vi "USB-HID-LabVIEW.vi"() -> ()   [LabVIEW 2016]
uses:
  <vilib>/Instr/_visa.llb/Select Event Type.ctl
panel:
  out "VISA resource name 2":refnum<visa-resource-name>
  out "error out":errorcluster
  out "string":string
  out "element":u8
  out "unsigned 8bit integer":u8[](array[numeric])
  out "status":bool
  in  "timeout (0)":u32
  in  "number":u8
  in  "error in (no error)":errorcluster
  in  "VISA resource name":refnum<visa-resource-name>
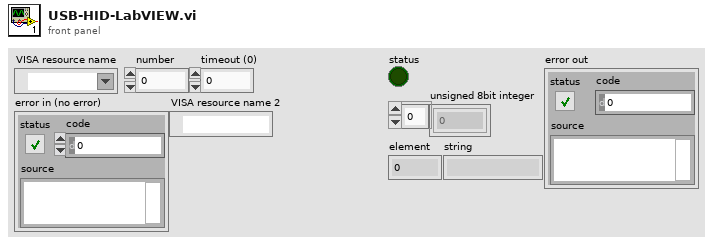
[diagram p1: front panel]
types:
  T1 = typedef "Select Event Type.ctl" = u32
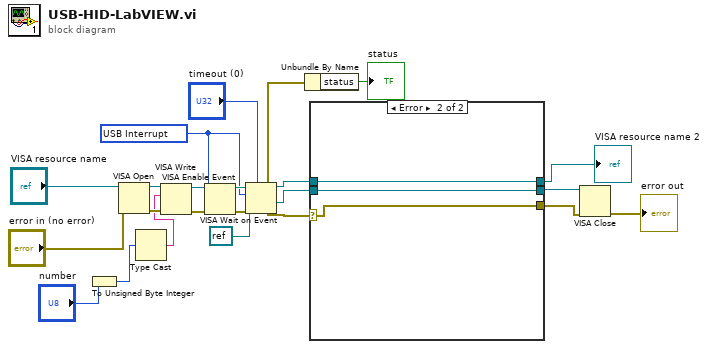
[diagram p0: block diagram]
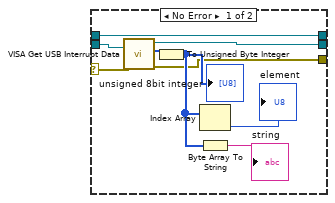
[diagram p2: hidden frame]
diagram:
  w11 = T1 1073684535 items=["Service Request"=1073684491, "Trigger"=3221168138, "Clear"=1073684493, "VXI Signal"=1073684512, "VXI/VME Interrupt"=3221168161, "VXI/VME Sysfail"=1073684509, "VXI/VME Sysreset"=1073684510, "GPIB CIC"=1073684498, "GPIB Talk"=1073684499, "GPIB Listen"=1073684500, "PXI Interrupt"=1073684514, "Serial Break"=1073684515, "Serial TermChar"=1073684516, "Serial CTS"=1073684521, "Serial DSR"=1073684522, "Serial DCD"=1073684524, "Serial RI"=1073684526, "Serial Character"=1073684533, "USB Interrupt"=1073684535, "All Enabled"=1073709055] ("Event Type")
  n1 = To Unsigned Byte Integer(number="number") -> (unsigned 8bit integer=w15:u8)
  n2 = VISA Open(error in (no error)="error in (no error)", VISA resource name="VISA resource name") -> (VISA resource name=w19:refnum<visa-resource-name>, error out=w20:errorcluster)  [unwired: 3 in]
  n3 = Type Cast(x=w15) -> (*(type *) &x=w16:string)  [unwired: 1 in]
  n4 = VISA Write(VISA resource name=w19, write buffer=w16, error in (no error)=w20) -> (VISA resource name out=w17:refnum<visa-resource-name>, error out=w18:errorcluster)  [unwired: 1 out]
  n5 = VISA Enable Event(8:w18, 10:w11, 11:w17) -> (0:w13:errorcluster, 3:w12:refnum<visa-resource-name>)  [unwired: 1 in]
  n6 = VISA Wait on Event(7:"timeout (0)", 8:w13, 9:refnum<visa-resource-name> refnum ("event class (Generic Event)"), 10:w11, 11:w12) -> (0:w6:errorcluster, 1:w8:refnum<visa-resource-name>, 3:w7:refnum<visa-resource-name>)  [unwired: 1 out]
  n7 = Unbundle By Name(w6) -> ("status"=→"status":bool)
  n8 = case shown="Error" w6 {
    selector: w6 -> [w31 w32]
    tunnel: w8 -> [w30 w33]
    tunnel: [w29 w34] -> w1
    tunnel: w7 -> [w29 w34]
    tunnel: [w28 w33] -> w3
    tunnel: [w23 w32] -> w4
    frame No Error {
      n9 = call <vilib>:"VISA Get USB Interrupt Data.vi"("error in (no error)"=w31, "VISA USB Intr Event"=w30) -> ("error out"=w23:errorcluster, "data buffer"=w27:u8[], "VISA USB Intr Event out"=w28:refnum<visa-resource-name>)  [unwired: 7 in]
      n10 = To Unsigned Byte Integer(number=w27) -> (unsigned 8bit integer=w25:u8[])
      "unsigned 8bit integer" <- w25
      n11 = Index Array(array=w25) -> (element=→"element":u8)  [unwired: 1 in]
      n12 = Byte Array To String(unsigned byte array=w25) -> (string=→"string":string)
    }
    frame Error {
    }
  }
  "VISA resource name 2" <- w1
  n13 = VISA Close(VISA resource name=w3, error in (no error)=w4) -> (error out=→"error out":errorcluster)
